vi "Find Dynamic Dispatch Methods.vi"(8 "error in (no error)":errorcluster, 10 "Class Path":path) -> (0 "error out":errorcluster, 2 "Dynamic Dispatch VIs":path[](array[path]))   [LabVIEW 2020, in "_Mock Class Generator Test.lvclass"]
uses:
  _Mock Class Generator Test.lvclass
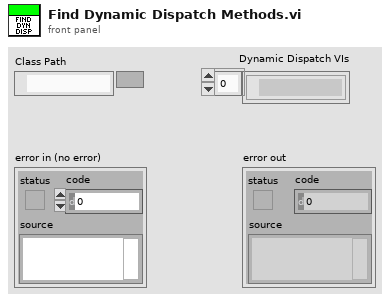
[diagram p1: front panel]
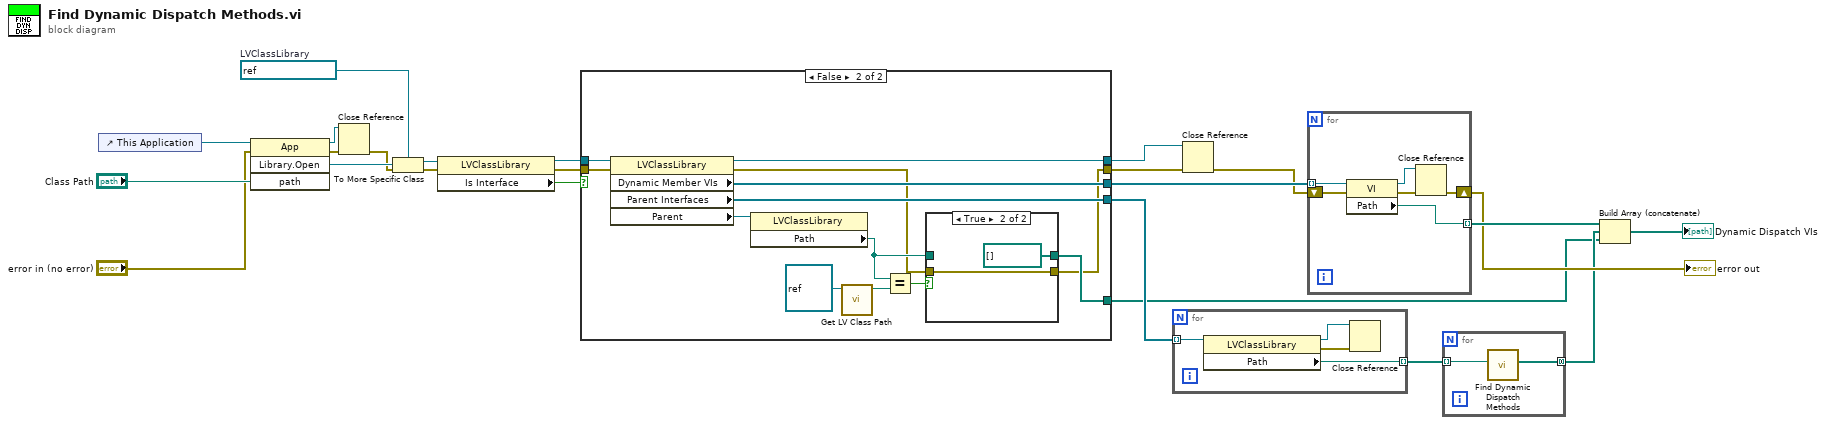
[diagram p0: block diagram]
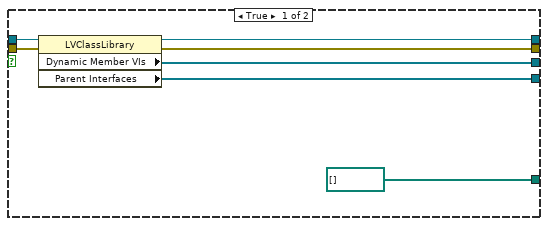
[diagram p2: hidden frame]
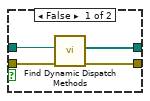
[diagram p3: hidden frame]
diagram:
  w20 = refnum<vi> refnum  # LVClassLibrary
  n1 = control-ref of="This Application"() -> (w24:refnum<vi>)
  n2 = invoke class="App" method="Library.Open"(reference=w24, error in="error in (no error)", "path"="Class Path") -> (reference out=w16:refnum<vi>, error out=w21:errorcluster, "Open Library"=w22:refnum<vi>)  [unwired: 1 in, 1 out]
  n3 = Close Reference(reference=w16, error in (no error)=w21) -> (error out=w17:errorcluster)
  n4 = To More Specific Class(target class=w20, reference=w22, error in=w17) -> (specific class reference=w4:refnum<vi>, error out=w19:errorcluster)
  n5 = property class="LVClassLibrary"(reference=w4, error in=w19) -> (reference out=w3:refnum<vi>, error out=w5:errorcluster, "Is Interface"=w2:bool)
  n6 = case shown="False" w2 {
    tunnel: [w31 w44] -> w15
    tunnel: [w30 w33] -> w13
    tunnel: [w29 w43] -> w10
    tunnel: [w28 w40] -> w9
    tunnel: w5 -> [w27 w42]
    tunnel: w3 -> [w26 w41]
    tunnel: [path[] [] ("Dynamic Dispatch VIs") w38] -> w1
    frame True {
      n7 = property class="LVClassLibrary"(reference=w26, error in=w27) -> (reference out=w29:refnum<vi>, error out=w30:errorcluster, "Dynamic Member VIs"=w31:refnum<vi>[], "Parent Interfaces"=w28:refnum<vi>[])
    }
    frame False {
      n8 = property class="LVClassLibrary"(reference=w41, error in=w42) -> (reference out=w43:refnum<vi>, error out=w34:errorcluster, "Dynamic Member VIs"=w44:refnum<vi>[], "Parent Interfaces"=w40:refnum<vi>[], "Parent"=w39:refnum<vi>)
      n9 = property class="LVClassLibrary"(reference=w39) -> ("Path"=w37:path)  [unwired: 1 in, 2 out]
      n10 = call <vilib>:"Get LV Class Path.vi"("object"=refnum<class> refnum) -> ("class path"=w35:path)  [unwired: 9 in, 1 out]
      n11 = Equal?(x=w37, y=w35) -> (x = y?=w32:bool)
      n12 = case shown="True" w32 {
        tunnel: [w48 path[] [] ("Dynamic Dispatch VIs")] -> w38
        tunnel: w37 -> [w47 _]
        tunnel: w34 -> [w46 w49]
        tunnel: [w45 w49] -> w33
        frame False {
          n13 = call "Find Dynamic Dispatch Methods.vi"("error in (no error)"=w46, "Class Path"=w47) -> ("error out"=w45:errorcluster, "Dynamic Dispatch VIs"=w48:path[])  [unwired: 8 in]
        }
        frame True {
        }
      }
    }
  }
  n14 = for {
    tunnel: w9 -> [w54] mode=indexing
    tunnel: [w53] -> w8 mode=indexing
    n15 = property class="LVClassLibrary"(reference=w54) -> (reference out=w52:refnum<vi>, error out=w51:errorcluster, "Path"=w53:path)  [unwired: 1 in]
    n16 = Close Reference(reference=w52, error in (no error)=w51) -> ()  [unwired: 1 out]
  }
  n17 = Close Reference(reference=w10, error in (no error)=w13) -> (error out=w11:errorcluster)
  n18 = for {
    tunnel: w15 -> [w60] mode=indexing
    tunnel: [w59] -> w14 mode=indexing
    shift-right: [w55] -> w12
    shift-left: w11 -> [w58]
    n19 = property class="VI"(reference=w60, error in=w58) -> (reference out=w56:refnum<vi>, error out=w57:errorcluster, "Path"=w59:path)
    n20 = Close Reference(reference=w56, error in (no error)=w57) -> (error out=w55:errorcluster)
  }
  "error out" <- w12
  n21 = for {
    tunnel: w8 -> [w62] mode=indexing
    tunnel: [w61] -> w6 mode=concatenating
    n22 = call "Find Dynamic Dispatch Methods.vi"("Class Path"=w62) -> ("Dynamic Dispatch VIs"=w61:path[])  [unwired: 9 in, 1 out]
  }
  n23 = Build Array (concatenate)(w14, w6, w1) -> (→"Dynamic Dispatch VIs":path[])
